vi "Get Run In Test Settings.vi"(11 "Model in":refnum<class "Model.lvclass">) -> (2 "Run In Test Settings":T1 {"Hold Time (s)" format="%.4f"}, 3 "Model out":refnum<class "Model.lvclass">)   [LabVIEW 2016, in "Model.lvclass"]
uses:
  Model.lvclass
  Typedefs/RunInSettings.ctl
  Model.lvclass/Model.ctl
  Typedefs/FAMT Typedefs.lvlib
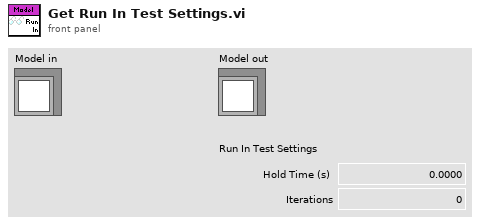
[diagram p1: front panel]
types:
  T1 = typedef "FAMT Typedefs.lvlib/RunInSettings.ctl" = cluster{"Hold Time (s)":dbl, "Iterations":i32}
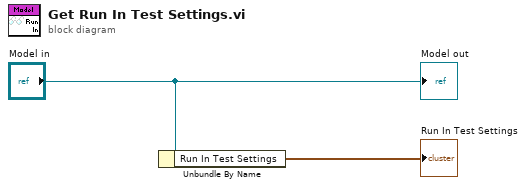
[diagram p0: block diagram]
diagram:
  n1 = Unbundle By Name("Model in") -> ("Run In Test Settings"=→"Run In Test Settings":T1)
  "Model out" <- "Model in"
